vi "DAQ_shutter_init.vi"(3 "error in":errorcluster, 5 "DAQ Settings":T1={"Shutters Settings"=[{"Name"="Shutter 1", "DAQ Channel/line"="Dev1/port0/line0", "Active"=FALSE}, {"Name"="Shutter 2", "DAQ Channel/line"="Dev1/port0/line1", "Active"=FALSE}], "Shutter Task"="", "Acquire Settings"=[], "AI Task"="", "Sample mode"=10178, "Number of Samples"=0, "Rate"=0.0, "AI Name"="", "DO Name"=""} {"Sample mode" items=["Finite Samples"=10178, "Continuous Samples"=10123, "Hardware Timed Single Point"=12522]; "Acquire Settings"."input terminal configuration" items=["default"=-1, "RSE"=10083, "NRSE"=10078, "Differential"=10106, "Pseudodifferential"=12529]}) -> (0 "error out":errorcluster, 2 "DO Task":refnum<k21>)   [LabVIEW 2019]
uses:
  Type defs/DAQ_set_Ctrl.ctl
  Type defs/DAQ_Shutter_Ctrl.ctl
  Type defs/DAQ_AI_Ctrl.ctl
  <vilib>/DAQmx/create/channels.llb/DAQmx Create Channel (DO-Digital Output).vi
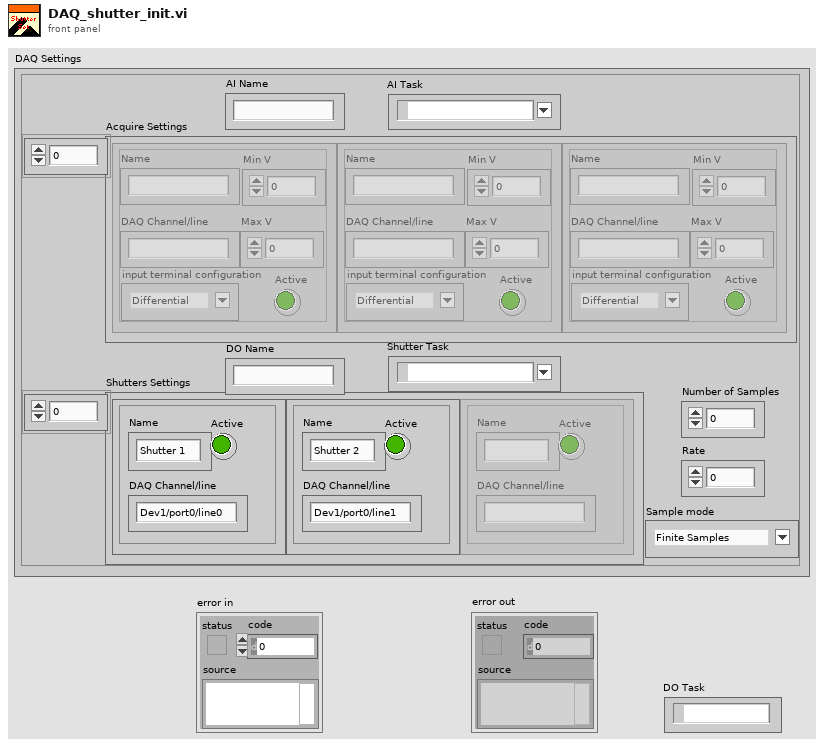
[diagram p1: front panel]
types:
  T1 = typedef "DAQ_set_Ctrl.ctl" = cluster{"Shutters Settings":T2[], "Shutter Task":refnum<k21>, "Acquire Settings":T3[], "AI Task":refnum<k21>, "Sample mode":i32, "Number of Samples":i32, "Rate":dbl, "AI Name":string, "DO Name":string}
  T2 = typedef "DAQ_Shutter_Ctrl.ctl" = cluster{"Name":string, "DAQ Channel/line":string, "Active":bool}
  T3 = typedef "DAQ_AI_Ctrl.ctl" = cluster{"Name":string, "DAQ Channel/line":string, "Max V":dbl, "Min V":dbl, "input terminal configuration":i32, "Active":bool}
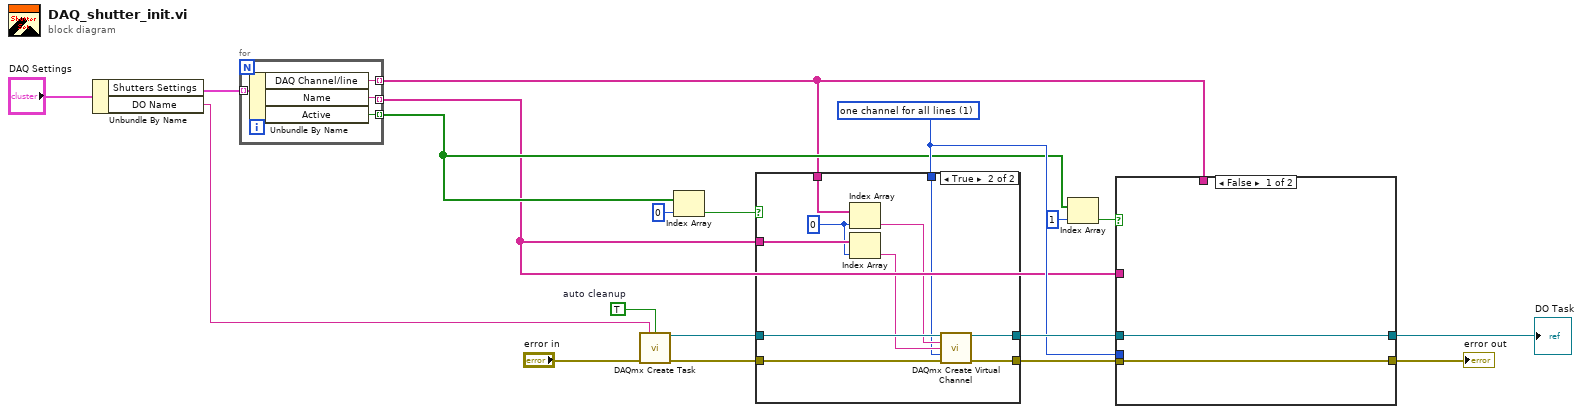
[diagram p0: block diagram]
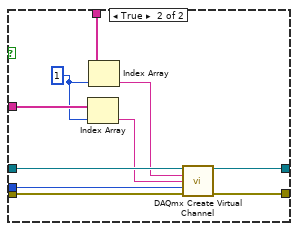
[diagram p2: hidden frame]
diagram:
  w12 = 1 items=["one channel for each line", "one channel for all lines"] ("line grouping")
  w18 = TRUE  # auto cleanup
  n1 = Unbundle By Name("DAQ Settings") -> ("Shutters Settings"=w7:T2[], "DO Name"=w5:string)
  n2 = for {
    tunnel: w7 -> [w23] mode=indexing
    tunnel: [w22] -> w2 mode=indexing
    tunnel: [w21] -> w3 mode=indexing
    tunnel: [w20] -> w4 mode=indexing
    n3 = Unbundle By Name(w23) -> ("DAQ Channel/line"=w22:string, "Name"=w21:string, "Active"=w20:bool)
  }
  n4 = call <vilib>:"DAQmx Create Task.vi"("new task name"=w5, "auto cleanup"=w18, "error in"="error in") -> ("task out"=w17:refnum<k21>, "error out"=w15:errorcluster)  [unwired: 11 in]
  n5 = Index Array(array=w4, index=0) -> (element=w10:bool)
  n6 = case shown="True" w10 {
    tunnel: w17 -> [w25 w35]
    tunnel: w3 -> [_ w34]
    tunnel: w2 -> [_ w33]
    tunnel: [w25 w31] -> w16
    tunnel: w15 -> [w24 w30]
    tunnel: [w24 w27] -> w14
    tunnel: w12 -> [_ w26]
    frame False {
    }
    frame True {
      w32 = 0 ("index")
      n7 = Index Array(array=w33, index=w32) -> (element=w29:string)
      n8 = Index Array(array=w34, index=w32) -> (element=w28:string)
      n9 = call-poly <vilib>:"DAQmx Create Virtual Channel.vi"("task in"=w35, "lines"=w29, "name to assign"=w28, "line grouping"=w26, "error in"=w30) -> ("task out"=w31:refnum<k21>, "error out"=w27:errorcluster)  [unwired: 9 in]
    }
  }
  n10 = Index Array(array=w4, index=1) -> (element=w8:bool)
  n11 = case shown="False" w8 {
    tunnel: w3 -> [_ w47]
    tunnel: w2 -> [_ w46]
    tunnel: w16 -> [w37 w44]
    tunnel: [w37 w43] -> w1
    tunnel: w14 -> [w36 w42]
    tunnel: [w36 w41] -> w13
    tunnel: w12 -> [_ w40]
    frame False {
    }
    frame True {
      w45 = 1 ("index")
      n12 = Index Array(array=w47, index=w45) -> (element=w39:string)
      n13 = Index Array(array=w46, index=w45) -> (element=w38:string)
      n14 = call-poly <vilib>:"DAQmx Create Virtual Channel.vi"("task in"=w44, "lines"=w38, "name to assign"=w39, "line grouping"=w40, "error in"=w42) -> ("task out"=w43:refnum<k21>, "error out"=w41:errorcluster)  [unwired: 9 in]
    }
  }
  "error out" <- w13
  "DO Task" <- w1
